vi "Update Firmware Dialog.vi"(8 "error in (no error)":errorcluster) -> (0 "error out":errorcluster, 2 "Result":T1, 3 "Cancelled?":bool)   [LabVIEW 2017]
doc: "Use this template to create a dialog box with event handling."
uses:
  <vilib>/SLSC/SLSC.lvlib
panel:
  in  "firmware path":path
  in  "password":string
  in  "username":string="admin"
  in  "Cancel":bool
  in  "OK":bool
  # "Firmware Path"
  # "Username"
  # "Password"
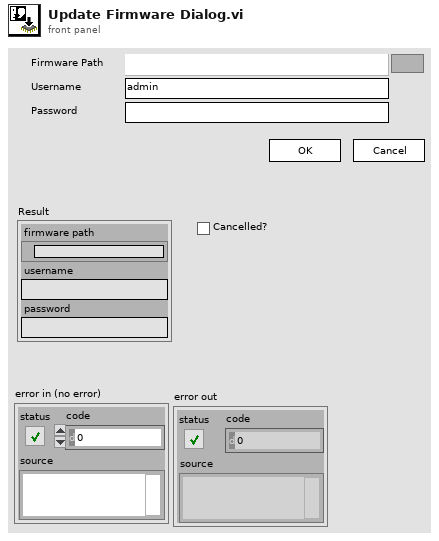
[diagram p1: front panel]
types:
  T1 = cluster{"firmware path":path, "username":string, "password":string}
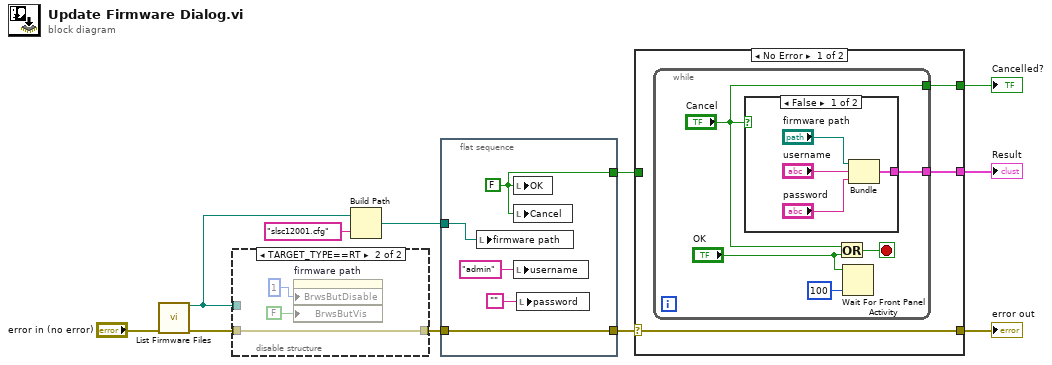
[diagram p0: block diagram]
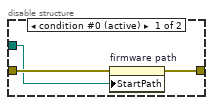
[diagram p2: hidden frame]
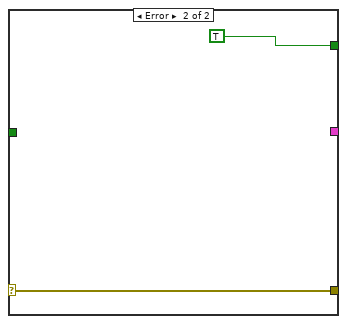
[diagram p4: hidden frame]
diagram:
  n1 = call <vilib>:"List Firmware Files.vi"("error in (no error)"="error in (no error)") -> ("default firmware path"=w3:path, "error out"=w6:errorcluster)  [unwired: 12 in, 1 out]
  n2 = disable-structure shown="TARGET_TYPE==RT" {
    disable-tunnel: w6 -> [w13 w15]
    disable-tunnel: [w14 w15] -> w5
    disable-tunnel: w3 -> [w12 _]
    frame condition #0 (active) {
      n3 = property on="firmware path" class="Path"(error in=w13, "StartPath"=w12) -> (error out=w14:errorcluster)  [unwired: 1 in, 1 out]
    }
    frame condition #1 {
      n4 = property on="firmware path" class="Path"("BrwsButDisable"=u8 1 ("Browse Button:Disabled"), "BrwsButVis"=FALSE ("Browse Button:Visible")) -> ()  [unwired: 2 in, 2 out]
    }
  }
  n5 = Build Path(base path=w3, name or relative path="slsc12001.cfg") -> (appended path=w2:path)
  n6 = flat-sequence {
    tunnel: [w21] -> w9
    tunnel: w2 -> [w19]
    tunnel: w5 -> [w18]
    tunnel: [w18] -> w4
    frame #0 {
      w21 = FALSE
      n7 = local write "firmware path"(w19) -> ()
      n8 = local write "OK"(w21) -> ()
      n9 = local write "Cancel"(w21) -> ()
      n10 = local write "username"("admin" ("username")) -> ()
      n11 = local write "password"("") -> ()
    }
  }
  n12 = case shown="No Error" w4 {
    selector: w4 -> [w25 w36]
    tunnel: [w25 w36] -> w11
    tunnel: [w23 TRUE] -> w10
    tunnel: [w24 _] -> w8
    tunnel: w9 -> [_ _]
    frame No Error {
      n13 = while {
        tunnel: [w30] -> w24
        tunnel: ["Cancel"] -> w23
        stop <- w28 stop-if-true
        n14 = case shown="False" "Cancel" {
          tunnel: [w32 _] -> w30
          frame False {
            n15 = Bundle("firmware path"="firmware path", "username"="username", "password"="password") -> (w32:T1)  [unwired: 1 in]
          }
          frame True {
          }
        }
        n16 = Or(x="Cancel", y="OK") -> (x .or. y?=w28:bool)
        n17 = Wait For Front Panel Activity(1:100 ("timeout ms (-1 never timeout)"), 3:"OK") -> ()  [unwired: 1 in, 1 out]
      }
    }
    frame Error {
    }
  }
  "Cancelled?" <- w10
  "Result" <- w8
  "error out" <- w11
